vi "runTestScenario.vi"(8 "error in (no error)":errorcluster, 11 "SSR_TTL High Test in":refnum<class "SSR_TTL High Test.lvclass">) -> (0 "error out":errorcluster, 2 "TestExecution":T1, 3 "SSR_TTL High Test out":refnum<class "SSR_TTL High Test.lvclass">)   [LabVIEW 2015, in "SSR_TTL High Test.lvclass"]
uses:
  SSR_TTL High Test.lvclass
  Typedefs/TestExecution.ctl
  Typedefs/WriteLogMessageInput.ctl
  Typedefs/TestScenarioTypes.ctl
  Typedefs/PassFailTest.ctl
  SSR_TTL High Test.lvclass/SSR_TTL High Test.ctl
  <userlib>/Common/ILC/ILC/ILC.lvclass/ILC.ctl
  Model/TestLog/ITestLog/ITestLog.lvclass
  Typedefs/ILCBTTypedefs.lvlib
  <userlib>/Common/ILC/ILC/ILC.lvclass
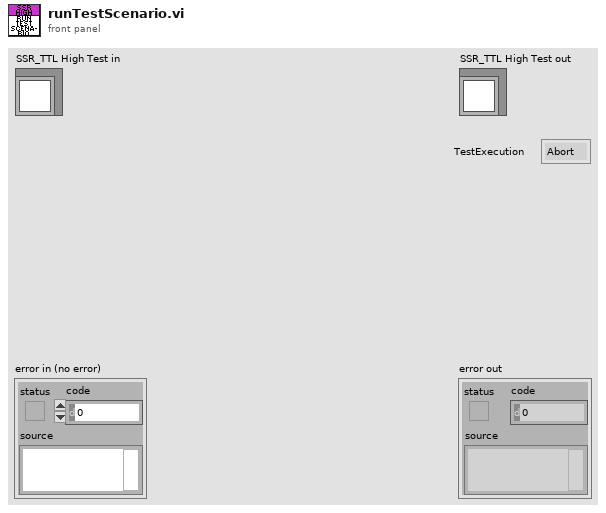
[diagram p1: front panel]
types:
  T1 = typedef "ILCBTTypedefs.lvlib/TestExecution.ctl" = enum16{"Abort", "Continue"}
  T2 = typedef "ILCBTTypedefs.lvlib/WriteLogMessageInput.ctl" = cluster{"Test Scenario":T3, "Description":string, "Actual Value":string, "Data File":string, "Result":T4}
  T3 = typedef "ILCBTTypedefs.lvlib/TestScenarioTypes.ctl" = enum16{"+3.3VA Supply Test", "+3.3VD Supply Test", "+5VA Supply Test", "+5VD Supply Test", "Unique ID Test", "TEDS Status Test", "LIMSW1_TTL Low Test", "LIMSW1_TTL High Test", "LIMSW2_TTL Low Test", "LIMSW2_TTL High Test", "Tachometer Test", "SSR_TTL Low Test", "SSR_TTL High Test", "SM_CW Low Test", "SM_CW High Test", "SM_CCW Low Test", "SM_CCW High Test", "SM_GPI Low Test", "SM_GPI High Test", "CW Motion Without Limit Test", "CW Motion With Limit Test", "CW Motion With Limit Interruption Test", "CW Motion on CCW Limit Test", "CCW Motion Without Limit Test", "CCW Motion With Limit Test", "CCW Motion With Limit Interruption Test", "CCW Motion on CW Limit Test", "RS232-TXD Low Test", "RS232-TXD High Test", "RS232-RTS Low Test", "RS232-RTS High Test", "RS232-RXD Low Test", "RS232-RXD High Test", "RS232-CTS Low Test", "RS232-CTS High Test", "Out_SS Low Test", "Out_SS High Test", "Out_SDI Low Test", "Out_SDI High Test", "Out_SCLK Low Test", "Out_SCLK High Test", "Reset Low Test", "Reset High Test", "1 Channel ADC Test", "3 Channel ADC Test", "5 Channel ADC Test", "Vref Test", "ROT Test", "DAC1 Test", "DAC2 Test", "DAC3 Test", "DAC4 Test", "BIAS Test", "EXC1 Test", "EXC2 Test", "EXC3 Test", "EXC4 Test"}
  T4 = typedef "ILCBTTypedefs.lvlib/PassFailTest.ctl" = enum16{"Fail", "Pass", "NA"}
  T5 = typedef "ILCBTTypedefs.lvlib/Digital Signal Level.ctl" = enum16{"Low", "High"}
  T6 = typedef "ILCCommon.lvlib/ILCTypedefs.lvlib/OutputData.ctl" = cluster{"Step & Direction":i16, "Blower RPM":u8, "PWM (SSR)":u8, "Ch1":u16, "Ch2":u16, "Ch3":u16, "Ch4":u16}
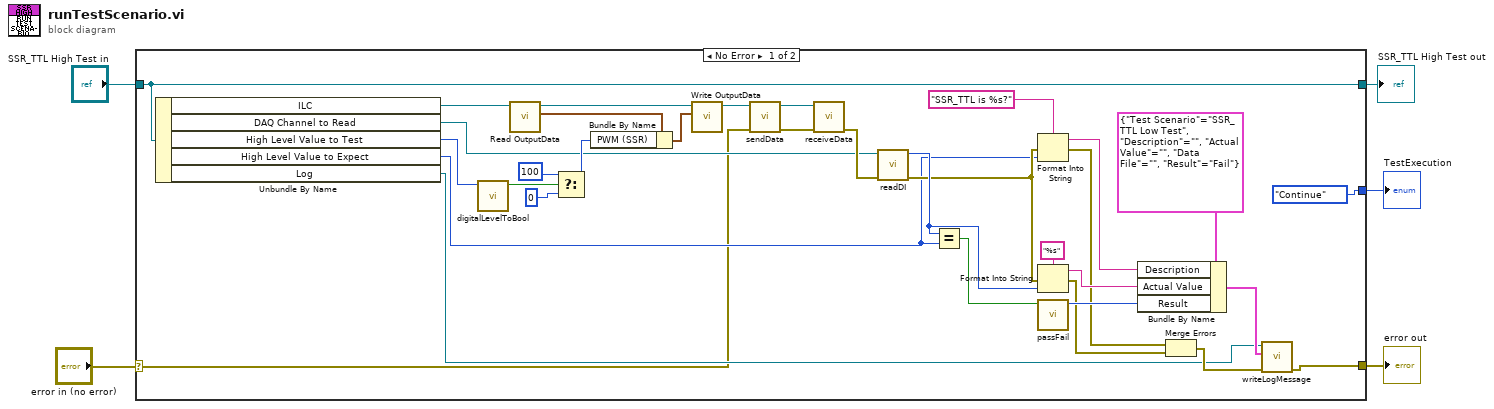
[diagram p0: block diagram]
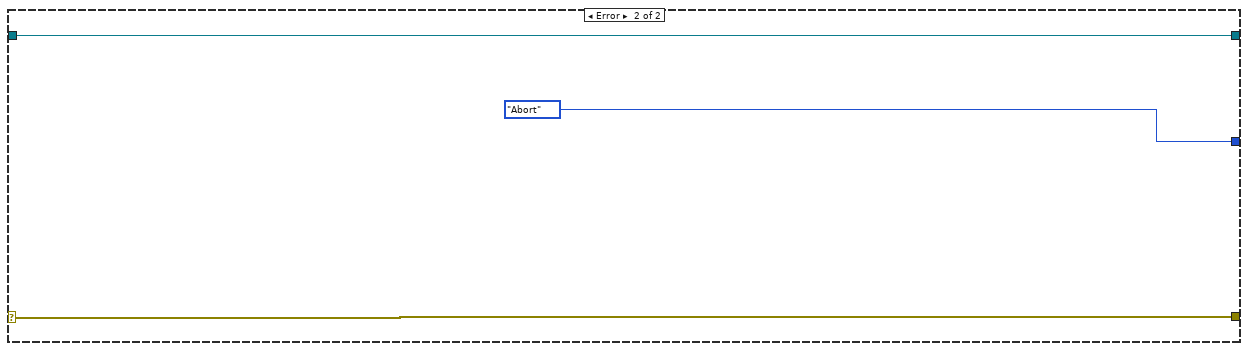
[diagram p2: hidden frame]
diagram:
  n1 = case shown="No Error" "error in (no error)" {
    selector: "error in (no error)" -> [w6 w40]
    tunnel: [w7 w40] -> w4
    tunnel: [w10 w41] -> w3
    tunnel: "SSR_TTL High Test in" -> [w10 w41]
    tunnel: [TestExecution."Continue" ("TestExecution") TestExecution."Abort" ("TestExecution")] -> w2
    frame No Error {
      n2 = Unbundle By Name(w10) -> ("ILC"=w20:refnum<class "ILC.lvclass">, "DAQ Channel to Read"=w18:refnum<k21>, "High Level Value to Test"=w19:T5, "High Level Value to Expect"=w12:T5, "Log"=w11:refnum<class "ITestLog.lvclass">)
      n3 = call "digitalLevelToBool.vi"("Digital Signal Level"=w19) -> ("Bool?"=w30:bool)  [unwired: 10 in]
      n4 = call <userlib>:"Read OutputData.vi"("ILC in"=w20) -> ("OutputData"=w31:T6, "ILC out"=w27:refnum<class "ILC.lvclass">)  [unwired: 9 in]
      n5 = Select(t=u8 100, s=w30, f=u8 0) -> (s? t:f=w29:u8)
      n6 = Bundle By Name(cluster=w31, "PWM (SSR)"=w29) -> (w28:T6)
      n7 = call <userlib>:"Write OutputData.vi"("OutputData"=w28, "ILC in"=w27) -> ("ILC out"=w24:refnum<class "ILC.lvclass">)  [unwired: 9 in]
      n8 = call <userlib>:"sendData.vi"("error in (no error)"=w6, "ILC in"=w24) -> ("error out"=w22:errorcluster, "ILC out"=w23:refnum<class "ILC.lvclass">)  [unwired: 8 in]
      n9 = call <userlib>:"receiveData.vi"("error in (no error)"=w22, "ILC in"=w23) -> ("error out"=w21:errorcluster)  [unwired: 8 in, 1 out]
      n10 = call "readDI.vi"("error in (no error)"=w21, "DAQ Channel To Read"=w18) -> ("error out"=w16:errorcluster, "Digital Signal Level"=w35:T5)  [unwired: 8 in]
      n11 = Equal?(x=w35, y=w12) -> (x = y?=w36:bool)
      n12 = Format Into String(format string="SSR_TTL is %s?", error in=w16, w12) -> (resulting string=w17:string, error out=w13:errorcluster)  [unwired: 1 in]
      n13 = Format Into String(format string="%s", error in=w16, w35) -> (resulting string=w33:string, error out=w14:errorcluster)  [unwired: 1 in]
      n14 = call "passFail.vi"("Boolean"=w36) -> ("Result"=w37:T4)  [unwired: 10 in]
      n15 = Bundle By Name(cluster=T2 {"Test Scenario"=enum."SSR_TTL Low Test", "Description"="", "Actual Value"="", "Data File"="", "Result"=enum."Fail"} ("WriteLogMessageInput"), "Description"=w17, "Actual Value"=w33, "Result"=w37) -> (w32:T2)
      n16 = Merge Errors(w13, w14) -> (w15:errorcluster)
      n17 = call-dynamic "writeLogMessage.vi"("error in (no error)"=w15, "WriteLogMessageInput"=w32, "ITestLog in"=w11) -> ("error out"=w7:errorcluster)  [unwired: 7 in, 1 out]
    }
    frame Error {
    }
  }
  "error out" <- w4
  "SSR_TTL High Test out" <- w3
  "TestExecution" <- w2
